vi "BG_corrSD.vi"(1 "Data":dbl[][](array[numeric]), 2 "upper pixel":dbl, 3 "lower pixel":dbl) -> (0 "Data corrected":dbl[][](array[numeric]))   [LabVIEW 2015]
uses:
  <vilib>/Analysis/NI_AALPro.lvlib
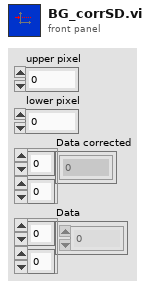
[diagram p1: front panel]
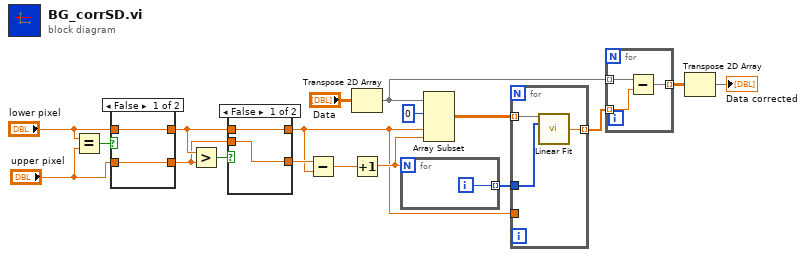
[diagram p0: block diagram]
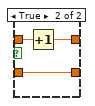
[diagram p2: hidden frame]
diagram:
  n1 = Equal?(x="lower pixel", y="upper pixel") -> (x = y?=w8:bool)
  n2 = case shown="False" w8 {
    tunnel: [w20 w22] -> w6
    tunnel: "lower pixel" -> [w20 w23]
    tunnel: [w19 w21] -> w4
    tunnel: "upper pixel" -> [w19 w21]
    frame False {
    }
    frame True {
      n3 = Increment(x=w23) -> (x+1=w22:dbl)
    }
  }
  n4 = Greater?(x=w6, y=w4) -> (0:w10:bool)
  n5 = case shown="False" w10 {
    tunnel: w6 -> [w24 w27]
    tunnel: [w25 w27] -> w11
    tunnel: w4 -> [w25 w26]
    tunnel: [w24 w26] -> w9
    frame False {
    }
    frame True {
    }
  }
  n6 = Subtract(x=w11, y=w9) -> (x-y=w13:dbl)
  n7 = Transpose 2D Array(2D array="Data") -> (transposed array=w18:dbl[][])
  n8 = Increment(x=w13) -> (x+1=w12:dbl)
  n9 = for {
    N: w12 -> [_]
    tunnel: [w28] -> w14 mode=indexing
    i -> [w28]
  }
  n10 = Array Subset(array=w18, index (row)=0 ("index"), index (col)=w9, length (col)=w12) -> (w15:dbl[][])  [unwired: 1 in]
  n11 = for {
    tunnel: w15 -> [w29] mode=indexing
    tunnel: [w31] -> w16 mode=indexing
    tunnel: w14 -> [w30]
    tunnel: w9 -> [_]
    n12 = call <vilib>:"Linear Fit.vi"("Y"=w29, "X"=w30) -> ("intercept"=w31:dbl)  [unwired: 9 in, 4 out]
  }
  n13 = for {
    tunnel: w18 -> [w34] mode=indexing
    tunnel: w16 -> [w33] mode=indexing
    tunnel: [w32] -> w3 mode=indexing
    n14 = Subtract(x=w34, y=w33) -> (x-y=w32:dbl[])
  }
  n15 = Transpose 2D Array(2D array=w3) -> (transposed array=→"Data corrected":dbl[][])
